vi "Listen for Connection.vi"(8 "error in (no error)":errorcluster, 11 "TCP Connection in":refnum<class "TCP Connection.lvclass">) -> (0 "error out":errorcluster, 2 "New Connection Made?":bool, 3 "TCP Connection out":refnum<class "TCP Connection.lvclass">)   [LabVIEW 2018, in "TCP Classes.lvlib" / "TCP Connection.lvclass"]
uses:
  TCP Connection.lvclass
  TCP Connection.lvclass/TCP Connection.ctl
  <vilib>/NI/STM/TCP/Write Meta Data (TCP Ref).vi
  <vilib>/NI/STM/TCP/Write Meta Data (TCP Clst).vi
  <vilib>/NI/STM/NI STM.lvlib
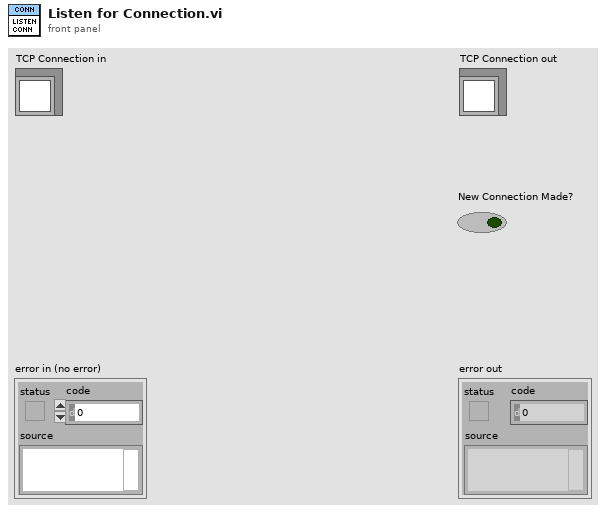
[diagram p1: front panel]
types:
  T1 = typedef "stm_MetaDataElement.ctl" = string
  T2 = typedef "NI STM.lvlib/TCP Connection Info.ctl" = cluster{"connection ID":refnum<k5>, "meta data":T3[]}
  T3 = typedef "NI STM.lvlib/MetaDataElement.ctl" = string
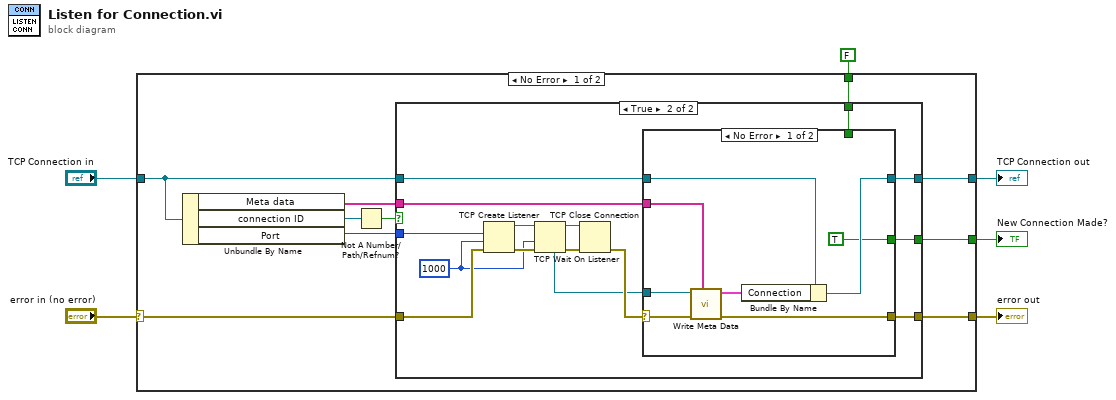
[diagram p0: block diagram]
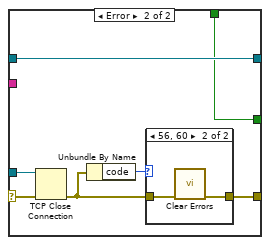
[diagram p3: hidden frame]
diagram:
  n1 = case shown="No Error" "error in (no error)" {
    selector: "error in (no error)" -> [w13 w55]
    tunnel: [w12 w55] -> w5
    tunnel: [w10 w54] -> w3
    tunnel: "TCP Connection in" -> [w11 w54]
    tunnel: [w8 w53] -> w2
    tunnel: FALSE ("Connection Made?") -> [w7 w53]
    frame No Error {
      n2 = Unbundle By Name(w11) -> ("Meta data"=w9:T1[], "connection ID"=w16:refnum<k5>, "Port"=w14:u16)
      n3 = Not A Number/Path/Refnum?(number/path/refnum=w16) -> (NaN/Path/Refnum?=w15:bool)
      n4 = case shown="True" w15 {
        tunnel: w14 -> [_ w30]
        tunnel: w13 -> [w18 w29]
        tunnel: [w18 w23] -> w12
        tunnel: w11 -> [w19 w25]
        tunnel: [w19 w24] -> w10
        tunnel: w9 -> [_ w22]
        tunnel: [w17 w21] -> w8
        tunnel: w7 -> [w17 w20]
        frame False {
        }
        frame True {
          w28 = 1000 ("timeout ms (wait forever: -1)")
          n5 = TCP Create Listener(8:w29, 9:w28, 10:w30) -> (0:w34:errorcluster, 3:w31:refnum<k5>)  [unwired: 2 in, 1 out]
          n6 = TCP Wait On Listener(8:w34, 9:w28, 11:w31) -> (0:w33:errorcluster, 3:w32:refnum<k5>, 4:w26:refnum<k5>)  [unwired: 1 in, 2 out]
          n7 = TCP Close Connection(connection ID=w32, error in (no error)=w33) -> (error out=w27:errorcluster)  [unwired: 1 in, 1 out]
          n8 = case shown="No Error" w27 {
            selector: w27 -> [w41 w48]
            tunnel: w26 -> [w42 w49]
            tunnel: w25 -> [w40 w47]
            tunnel: [w38 w47] -> w24
            tunnel: [w37 w43] -> w23
            tunnel: w22 -> [w36 _]
            tunnel: [TRUE ("Connection Made?") w46] -> w21
            tunnel: w20 -> [_ w46]
            frame No Error {
              n9 = call-poly <vilib>:"Write Meta Data.vi"("meta data"=w36, "error in"=w41, "connection ID"=w42) -> ("error out"=w37:errorcluster, "connection info out"=w39:T2)  [unwired: 7 in]
              n10 = Bundle By Name(cluster=w40, "Connection"=w39) -> (w38:refnum<class "TCP Connection.lvclass">)
            }
            frame Error {
              n11 = TCP Close Connection(connection ID=w49, error in (no error)=w48) -> (error out=w45:errorcluster)  [unwired: 1 in, 1 out]
              n12 = Unbundle By Name(w45) -> ("code"=w44:i32)
              n13 = case shown="56, 60" w44 {
                tunnel: w45 -> [w50 w52]
                tunnel: [w50 w51] -> w43
                frame 0, Default {
                }
                frame 56, 60 {
                  n14 = call <vilib>:"Clear Errors.vi"("error in (no error)"=w52) -> ("error out"=w51:errorcluster)  [unwired: 5 in, 1 out]
                }
              }
            }
          }
        }
      }
    }
    frame Error {
    }
  }
  "error out" <- w5
  "TCP Connection out" <- w3
  "New Connection Made?" <- w2
